vi "Generate HA yaml config.vi"() -> ()   [LabVIEW 2021]
uses:
  df90f6c2-59a7-465d-b42e-4f1643e906b5.vi
  <vilib>/Comparison/Less/Less Functor/Less Functor.lvclass
panel:
  out "Unhandled":string[](array[string])
  out "Yaml config":string
  in  "Global name":string[](array[string])=["IO", "MAIN"]
  out "Items":string[](array[string])
  in  "TwinCAT process image export file":path=path "C:/HomePLC/HomePLC-Example/Tools/Process image export.xml"
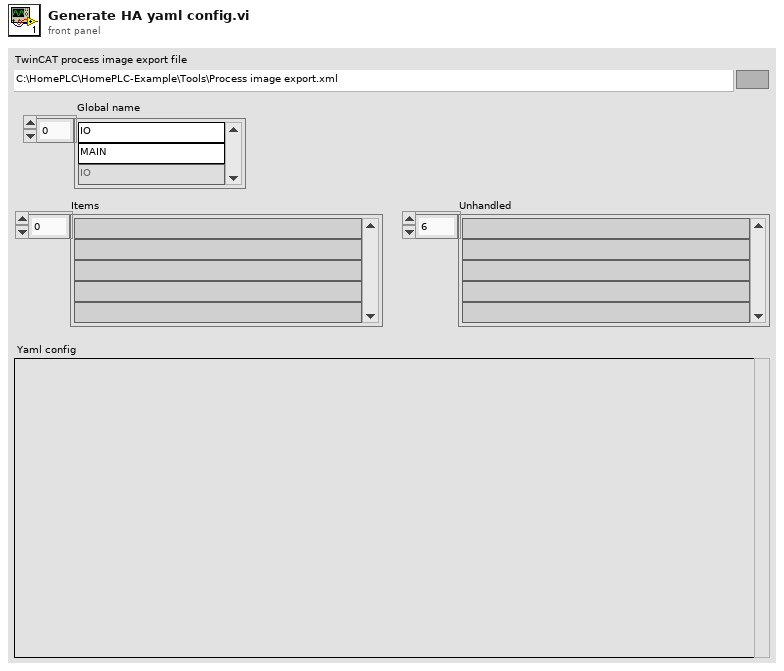
[diagram p1: front panel]
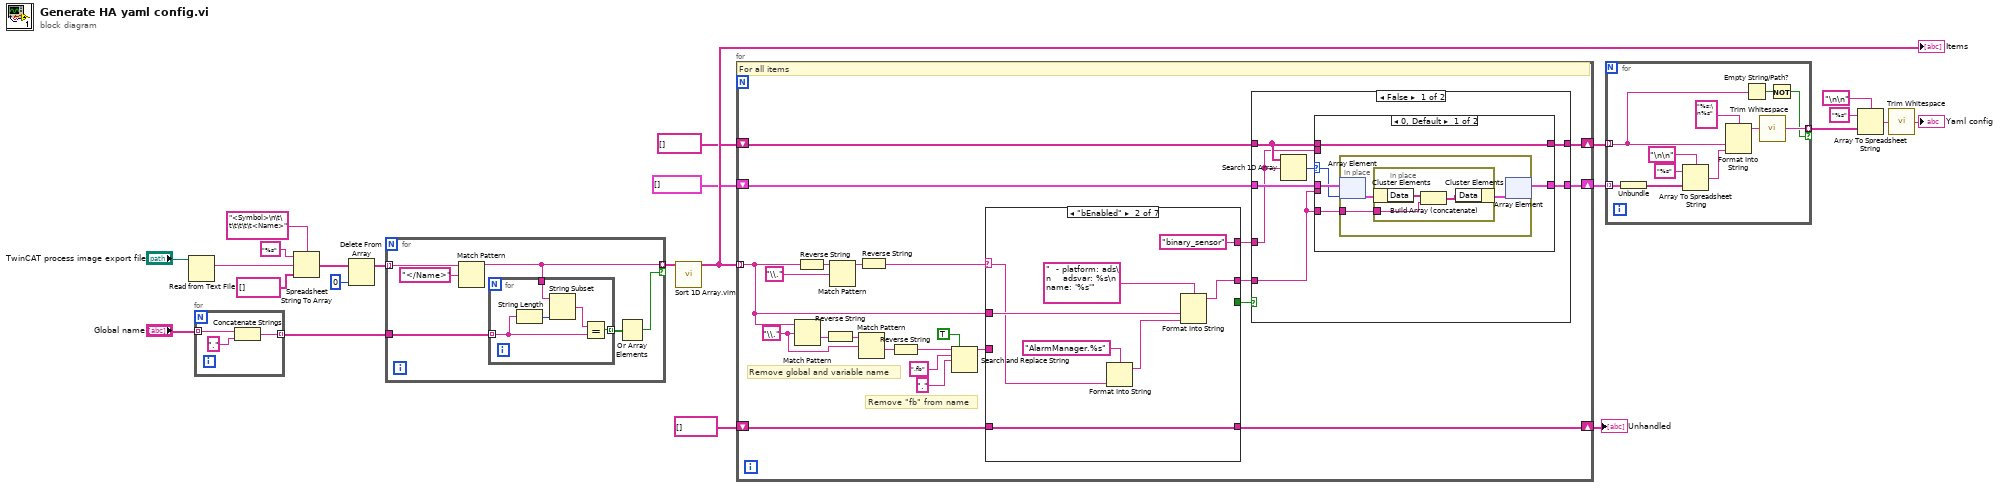
[diagram p0: block diagram]
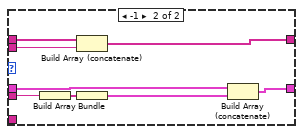
[diagram p2: hidden frame]
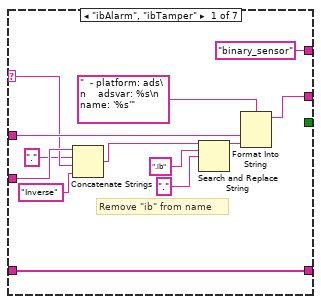
[diagram p4: hidden frame]
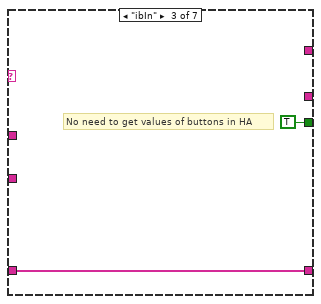
[diagram p5: hidden frame]
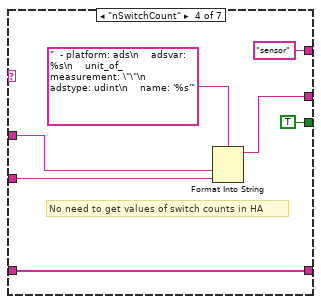
[diagram p6: hidden frame]
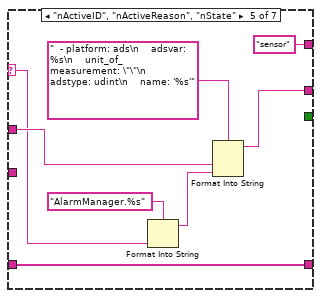
[diagram p7: hidden frame]
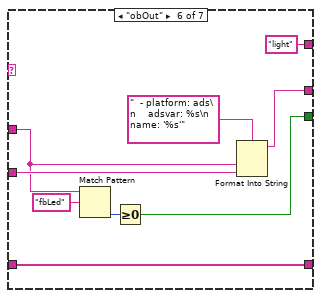
[diagram p8: hidden frame]
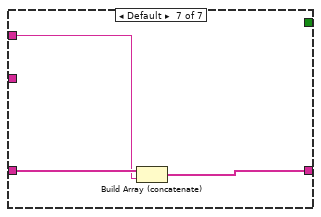
[diagram p9: hidden frame]
diagram:
  n1 = Read from Text File(file (use dialog)="TwinCAT process image export file") -> (text=w22:string)  [unwired: 3 in, 3 out]
  n2 = for {
    tunnel: "Global name" -> [w26] mode=indexing
    tunnel: [w24] -> w13 mode=indexing
    n3 = Concatenate Strings(w26, "." ("string")) -> (w24:string)
  }
  n4 = Spreadsheet String To Array(delimiter (Tab)="<Symbol>\n\t\t\t\t\t\t<Name>", format string="%s", spreadsheet string=w22, array type (2D Dbl)=string[] []) -> (array=w17:string[])
  n5 = Delete From Array(array=w17, index=0) -> (array with subset deleted=w16:string[])  [unwired: 1 in, 1 out]
  n6 = for {
    tunnel: w16 -> [w32] mode=indexing
    tunnel: [w29] -> w18 mode=indexing if=w27
    tunnel: w13 -> [w30]
    n7 = Match Pattern(string=w32, regular expression="</Name>") -> (before substring=w29:string)  [unwired: 1 in, 3 out]
    n8 = for {
      tunnel: w30 -> [w36] mode=indexing
      tunnel: w29 -> [w34]
      tunnel: [w33] -> w28 mode=indexing
      n9 = String Length(string=w36) -> (length=w37:i32)
      n10 = String Subset(string=w34, length (rest)=w37) -> (substring=w35:string)  [unwired: 1 in]
      n11 = Equal?(x=w35, y=w36) -> (x = y?=w33:bool)
    }
    n12 = Or Array Elements(Boolean array=w28) -> (logical OR=w27:bool)
  }
  n13 = call "Sort 1D Array.vim"("unsorted array"=w18) -> ("sorted array"=w12:string[])  [unwired: 10 in]
  "Items" <- w12
  n14 = for {
    tunnel: w12 -> [w49] mode=indexing
    shift-right: [w47] -> w9
    shift-left: string[] [] -> [w48]
    shift-right: [w45] -> w8
    shift-left: cluster{"Data":string[]}[] [] -> [w46]
    shift-right: [w39] -> w1
    shift-left: string[] [] -> [w40]
    w58 = "\\." ("regular expression")
    # "Remove \"fb\" from name"
    # "Remove global and variable name"
    # "For all items"
    n15 = Match Pattern(string=w49, regular expression=w58) -> (after substring=w60:string)  [unwired: 1 in, 3 out]
    n16 = Reverse String(1:w49) -> (0:w50:string)
    n17 = Reverse String(1:w60) -> (0:w59:string)
    n18 = Match Pattern(string=w50, regular expression="\\.") -> (before substring=w52:string)  [unwired: 1 in, 3 out]
    n19 = Match Pattern(string=w59, regular expression=w58) -> (after substring=w57:string)  [unwired: 1 in, 3 out]
    n20 = Reverse String(1:w52) -> (0:w43:string)
    n21 = Reverse String(1:w57) -> (0:w56:string)
    n22 = Search and Replace String(replace all?=TRUE ("replace all? (F)"), input string=w56, search string=".fb", replace string="." ("replace string (\"\")")) -> (result string=w55:string)  [unwired: 4 in, 3 out]
    n23 = case shown="\"bEnabled\"" w43 {
      selector: w43 -> [w93 w102 _ _ w120 _ _]
      tunnel: w49 -> [w98 w106 _ w117 w125 w131 w136]
      tunnel: [w100 w108 _ w115 w124 w134 _] -> w44
      tunnel: w55 -> [w94 _ _ w116 _ w133 _]
      tunnel: ["binary_sensor" ("format string") "binary_sensor" ("format string") _ "sensor" ("format string") "sensor" ("format string") "light" ("format string") _] -> w42
      tunnel: [_ _ TRUE TRUE _ w128 _] -> w41
      tunnel: w40 -> [w89 w105 w110 w112 w122 w127 w138]
      tunnel: [w89 w105 w110 w112 w122 w127 w137] -> w39
      frame "ibAlarm", "ibTamper" {
        # "Remove \"ib\" from name"
        n24 = Concatenate Strings(w94, "." ("string"), w93, "Inverse" ("string")) -> (w92:string)
        n25 = Search and Replace String(input string=w92, search string=".ib", replace string="." ("replace string (\"\")")) -> (result string=w95:string)  [unwired: 5 in, 3 out]
        n26 = Format Into String(format string="  - platform: ads\n    adsvar: %s\n    name: '%s'", w98, w95) -> (resulting string=w100:string)  [unwired: 2 in, 1 out]
      }
      frame "bEnabled" {
        n27 = Format Into String(format string="AlarmManager.%s", w102) -> (resulting string=w103:string)  [unwired: 2 in, 1 out]
        n28 = Format Into String(format string="  - platform: ads\n    adsvar: %s\n    name: '%s'", w106, w103) -> (resulting string=w108:string)  [unwired: 2 in, 1 out]
      }
      frame "ibIn" {
        # "No need to get values of buttons in HA"
      }
      frame "nSwitchCount" {
        # "No need to get values of switch counts in HA"
        n29 = Format Into String(format string="  - platform: ads\n    adsvar: %s\n    unit_of_measurement: \"\"\n    adstype: udint\n    name: '%s'", w117, w116) -> (resulting string=w115:string)  [unwired: 2 in, 1 out]
      }
      frame "nActiveID", "nActiveReason", "nState" {
        n30 = Format Into String(format string="AlarmManager.%s", w120) -> (resulting string=w121:string)  [unwired: 2 in, 1 out]
        n31 = Format Into String(format string="  - platform: ads\n    adsvar: %s\n    unit_of_measurement: \"\"\n    adstype: udint\n    name: '%s'", w125, w121) -> (resulting string=w124:string)  [unwired: 2 in, 1 out]
      }
      frame "obOut" {
        n32 = Match Pattern(string=w131, regular expression="fbLed") -> (offset past match=w129:i32)  [unwired: 1 in, 3 out]
        n33 = Greater Or Equal To 0?(x=w129) -> (x >= 0?=w128:bool)
        n34 = Format Into String(format string="  - platform: ads\n    adsvar: %s\n    name: '%s'", w131, w133) -> (resulting string=w134:string)  [unwired: 2 in, 1 out]
      }
      frame Default {
        n35 = Build Array (concatenate)(w138, w136) -> (w137:string[])
      }
    }
    n36 = case shown="False" w41 {
      tunnel: w48 -> [w66 w88]
      tunnel: [w65 w88] -> w47
      tunnel: w46 -> [w64 w87]
      tunnel: [w63 w87] -> w45
      tunnel: w44 -> [w62 _]
      tunnel: w42 -> [w61 _]
      frame False {
        n37 = Search 1D Array(1D array=w66, element=w61) -> (index of element=w67:i32)  [unwired: 1 in]
        n38 = case shown="0, Default" w67 {
          selector: w67 -> [w70 _]
          tunnel: w66 -> [w72 w86]
          tunnel: [w72 w85] -> w65
          tunnel: w61 -> [_ w84]
          tunnel: w62 -> [_ w81]
          tunnel: w64 -> [w71 w83]
          tunnel: [w69 w82] -> w63
          tunnel: w62 -> [w68 _]
          frame 0, Default {
            n39 = in-place {
              in-place-border: w68 -> [w73]
              n40 = in-place-array #1(w71, w70) -> (w75:cluster{"Data":string[]})
              n41 = in-place {
                in-place-border: w73 -> [w76]
                n42 = in-place-cluster #2(w75) -> ("Data"=w78:string[])
                n43 = Build Array (concatenate)(w78, w76) -> (w77:string[])
                n44 = in-place-cluster #2("Data"=w77) -> (w74:cluster{"Data":string[]})
              }
              n45 = in-place-array #1(w74) -> (w69:cluster{"Data":string[]}[])  [unwired: 1 out]
            }
          }
          frame -1 {
            n46 = Build Array(w81) -> (w80:string[])
            n47 = Build Array (concatenate)(w86, w84) -> (w85:string[])
            n48 = Bundle(w80) -> (w79:cluster{string[]})  [unwired: 1 in]
            n49 = Build Array (concatenate)(w83, w79) -> (w82:cluster{"Data":string[]}[])
          }
        }
      }
      frame True {
      }
    }
  }
  "Unhandled" <- w1
  n50 = for {
    tunnel: w9 -> [w139] mode=indexing
    tunnel: w8 -> [w149] mode=indexing
    tunnel: [w143] -> w5 mode=indexing if=w141
    n51 = Unbundle(w149) -> ("Data"=w146:string[])
    n52 = Array To Spreadsheet String(delimiter (Tab)="\n\n", array=w146, 3:"%s" ("format string")) -> (spreadsheet string=w140:string)
    n53 = Format Into String(format string="%s:\n%s", w139, w140) -> (resulting string=w145:string)  [unwired: 2 in, 1 out]
    n54 = Empty String/Path?(string/path=w139) -> (empty?=w142:bool)
    n55 = call <vilib>:"Trim Whitespace.vi"("string"=w145) -> ("trimmed string"=w143:string)  [unwired: 1 in]
    n56 = Not(x=w142) -> (.not. x?=w141:bool)
  }
  n57 = Array To Spreadsheet String(delimiter (Tab)="\n\n", array=w5, 3:"%s" ("format string")) -> (spreadsheet string=w4:string)
  n58 = call <vilib>:"Trim Whitespace.vi"("string"=w4) -> ("trimmed string"=→"Yaml config":string)  [unwired: 1 in]
